vi "MemoryDialog.vi"(8 "Error In":errorcluster, 10 "Slot 1 Configuration":T1, 11 "Channel Patterns In":string[](array[string])) -> (0 "Error Out":errorcluster, 2 "Cancelled?":bool, 3 "Channel Patterns Out":string[](array[string]))   [LabVIEW 2012]
uses:
  SlotConfiguration.ctl
  BankConfiguration.ctl
  driver/Public/Controls/Slot.ctl
  libs/LV-Utilities/LV-Utilities.lvlib
  driver/Keithley-7001.lvlib
panel:
  out "Bank D Name":string
  out "Bank D Channel Names":string[](array[string])
  in  "Bank D Channel Enabled":bool[](array[boolean])
  out "Bank C Name":string
  out "Bank C Channel Names":string[](array[string])
  in  "Bank C Channel Enabled":bool[](array[boolean])
  out "Bank B Name":string
  out "Bank B Channel Names":string[](array[string])
  in  "Bank B Channel Enabled":bool[](array[boolean])=[FALSE, FALSE, FALSE, FALSE, FALSE, FALSE, FALSE, FALSE, FALSE, FALSE]
  out "Bank A Name":string
  out "Bank A Channel Names":string[](array[string])
  in  "Bank A Channel Enabled":bool[](array[boolean])=[FALSE, FALSE, FALSE, FALSE, FALSE, FALSE, FALSE, FALSE, FALSE, FALSE]
  in  "NEXT MEMORY LOCATION":bool
  in  "PREVIOUS MEMORY LOCATION":bool
  in  "Memory Location (1-100)":u8=1 min=1 max=100 step=1
  out "Channel Pattern":string
  in  "STORE":bool
  in  "RESET":bool
  in  "CANCEL":bool
  in  "DONE":bool
  # "CHANNELS"
  # "MEMORY"
  # "Location"
  # "Channel Pattern"
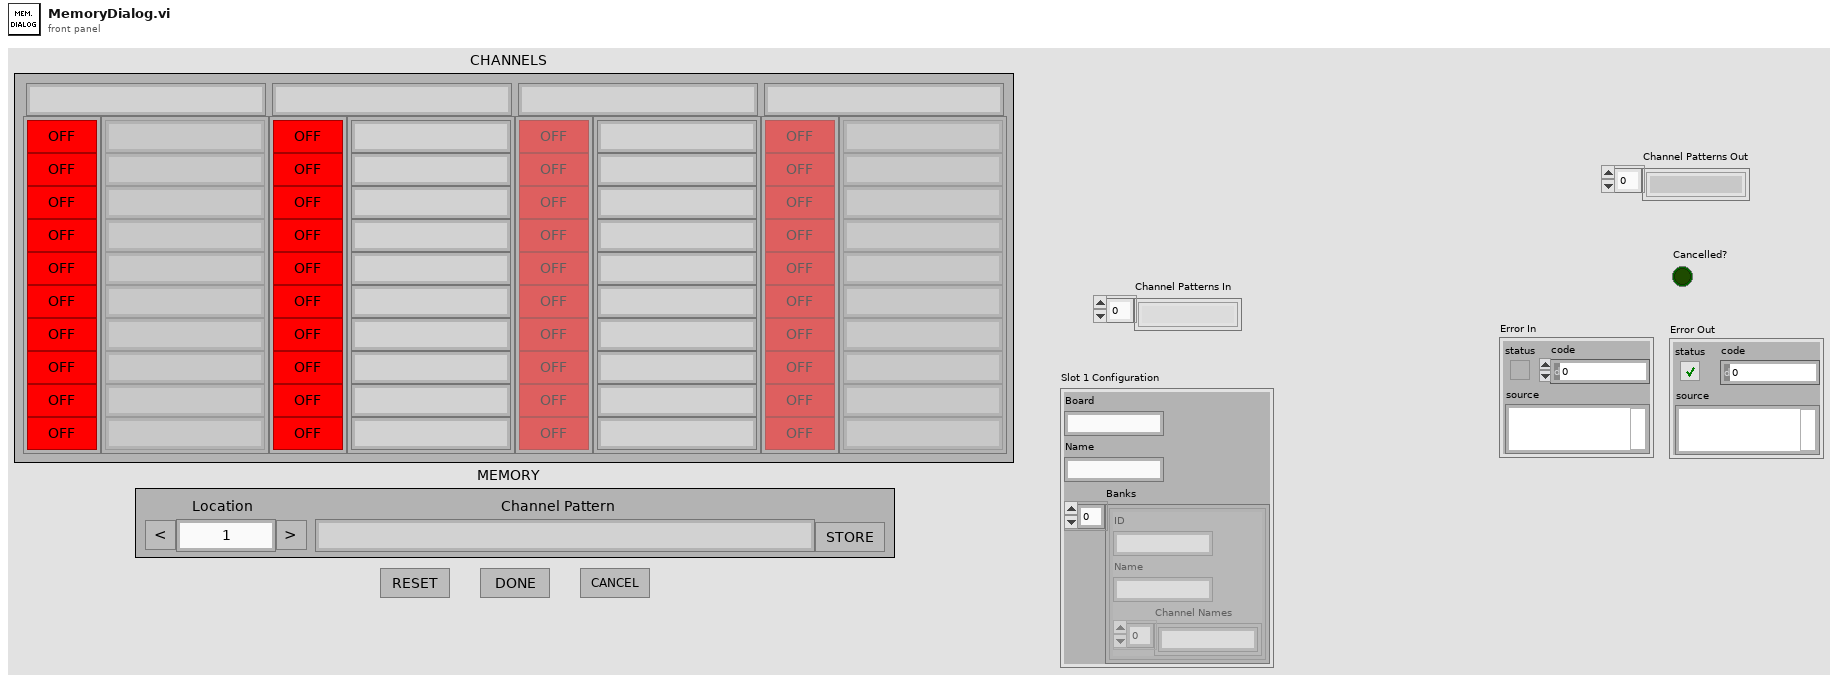
[diagram p1: front panel]
types:
  T1 = typedef "SlotConfiguration.ctl" = cluster{"Board":string, "Name":string, "Banks":T2[]}
  T2 = typedef "BankConfiguration.ctl" = cluster{"ID":string, "Name":string, "Channel Names":string[]}
  T3 = typedef "Keithley-7001.lvlib/Slot.ctl" = enum16{"Slot 1", "Slot 2"}
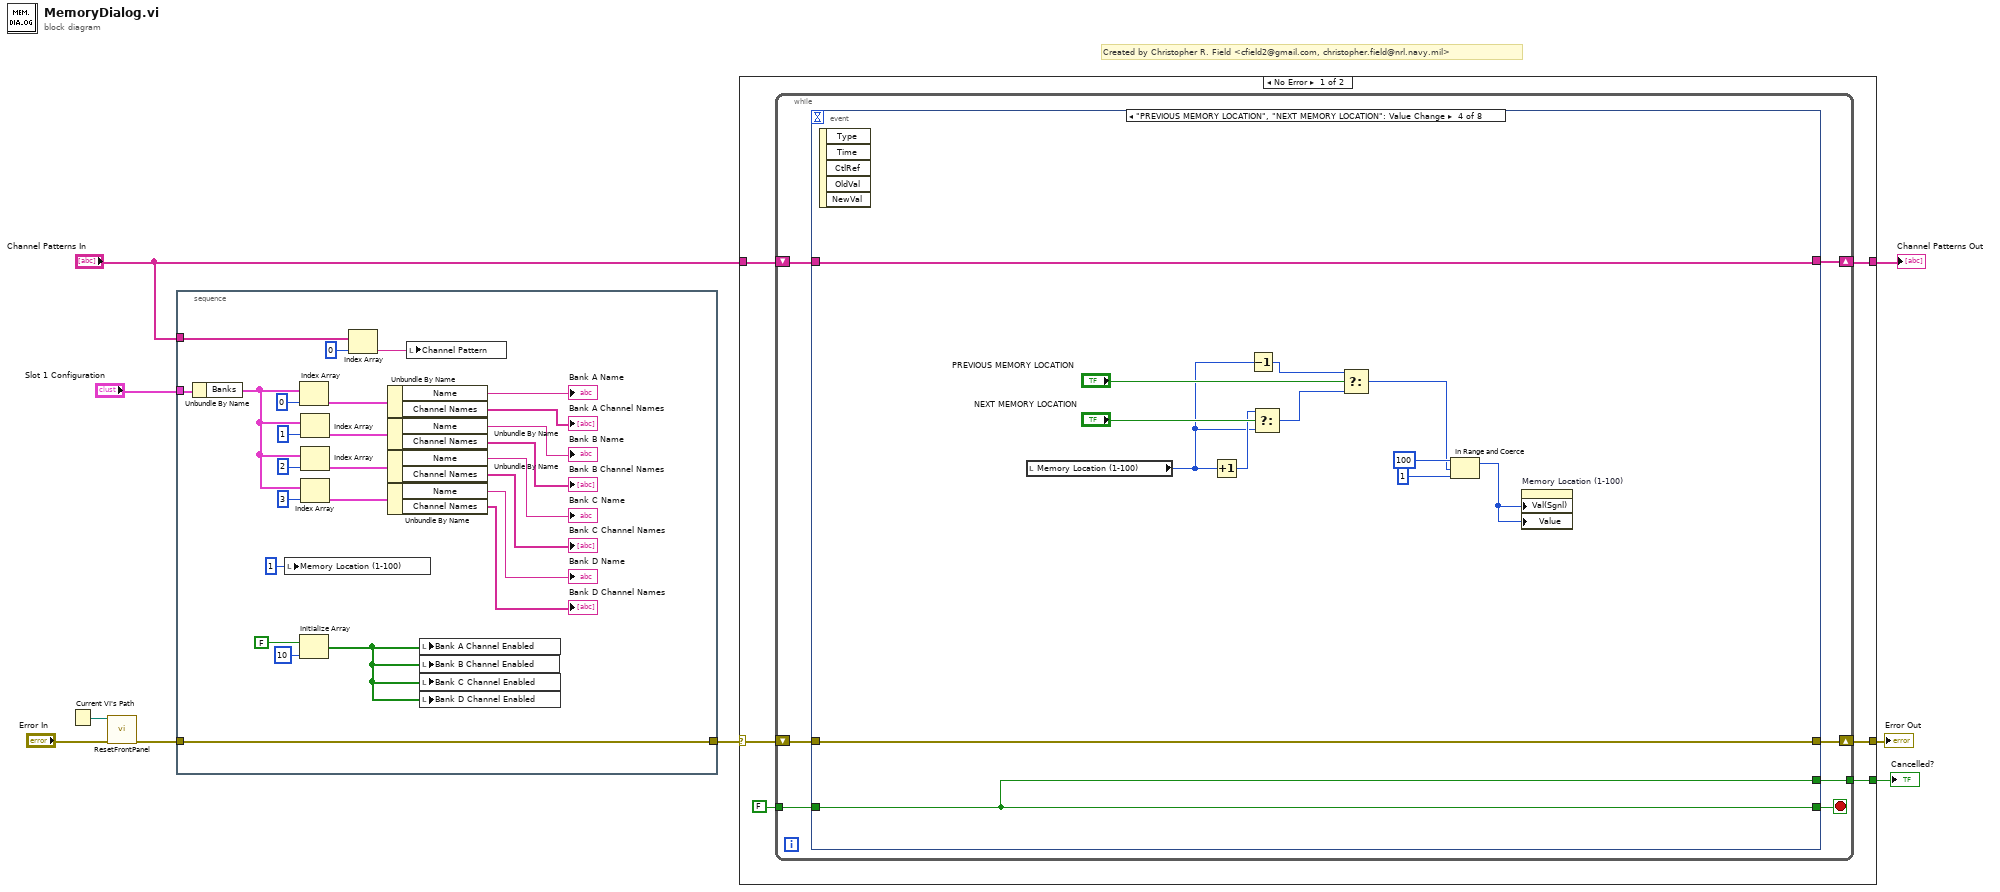
[diagram p0: block diagram]
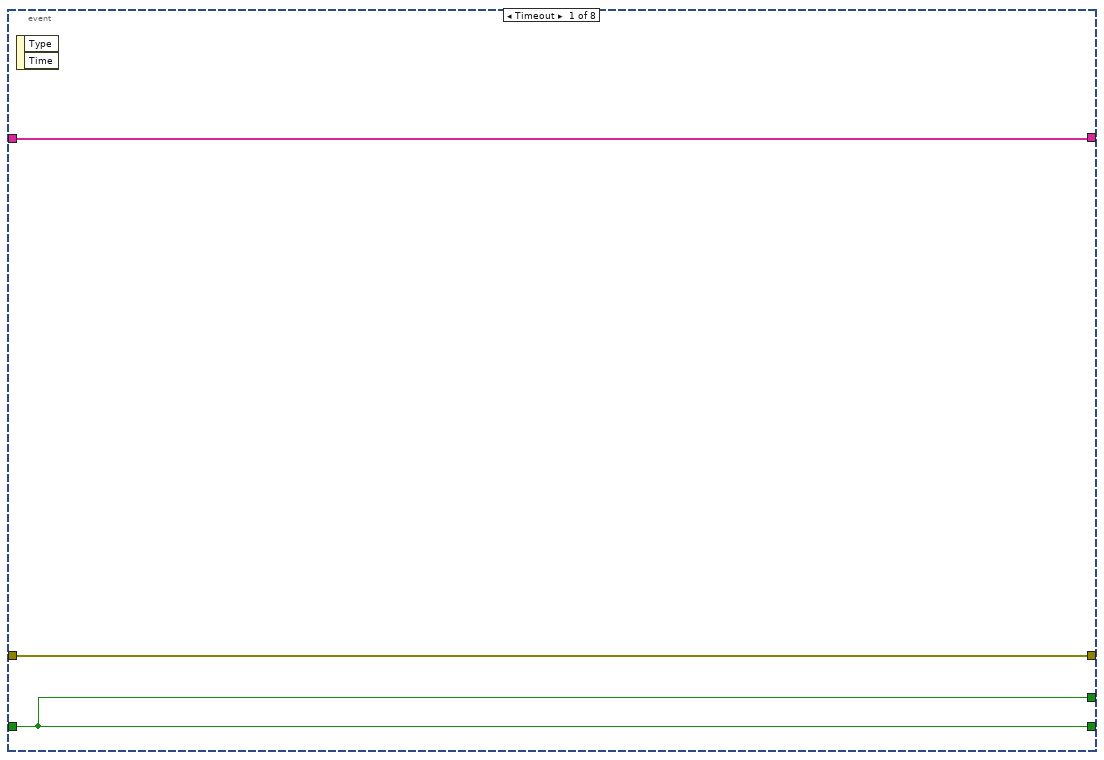
[diagram p2: hidden frame]
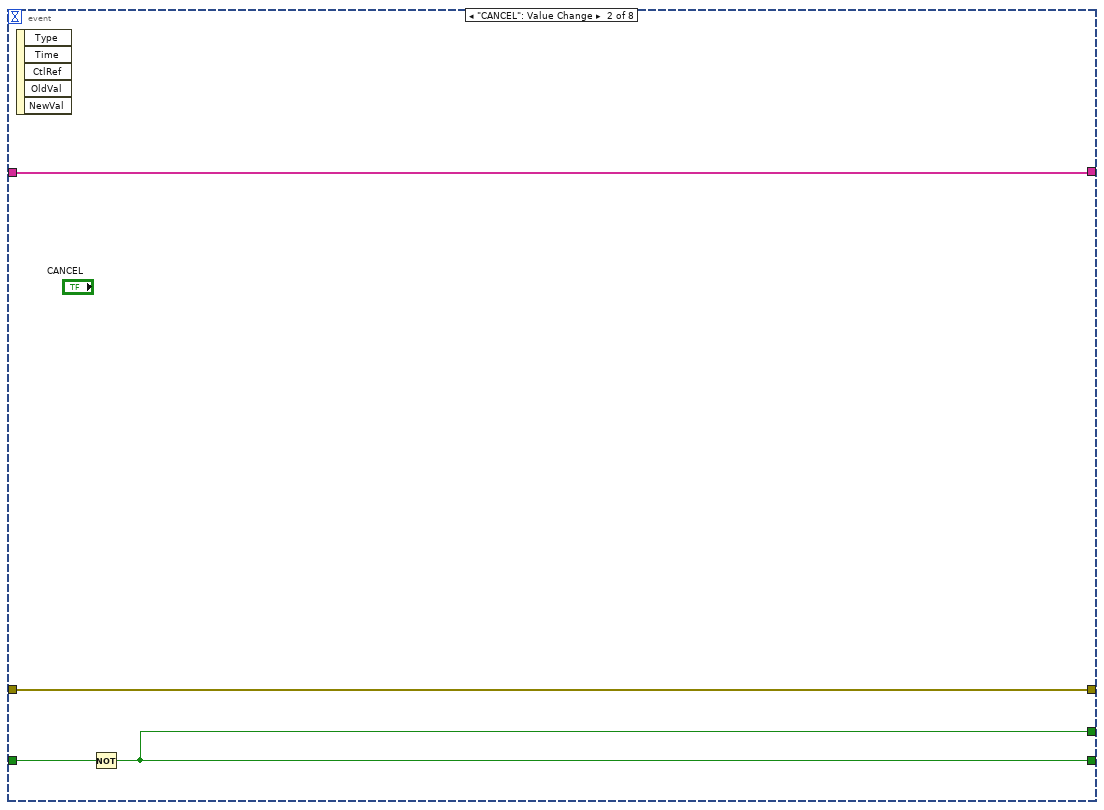
[diagram p3: hidden frame]
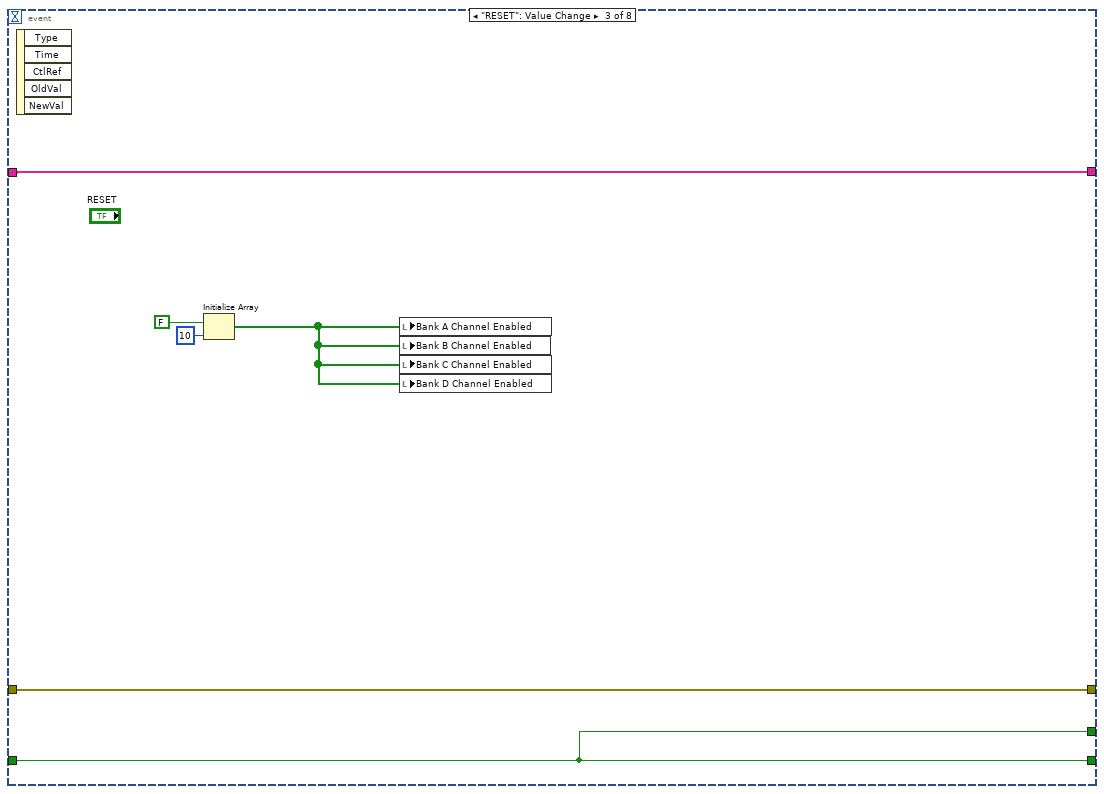
[diagram p4: hidden frame]
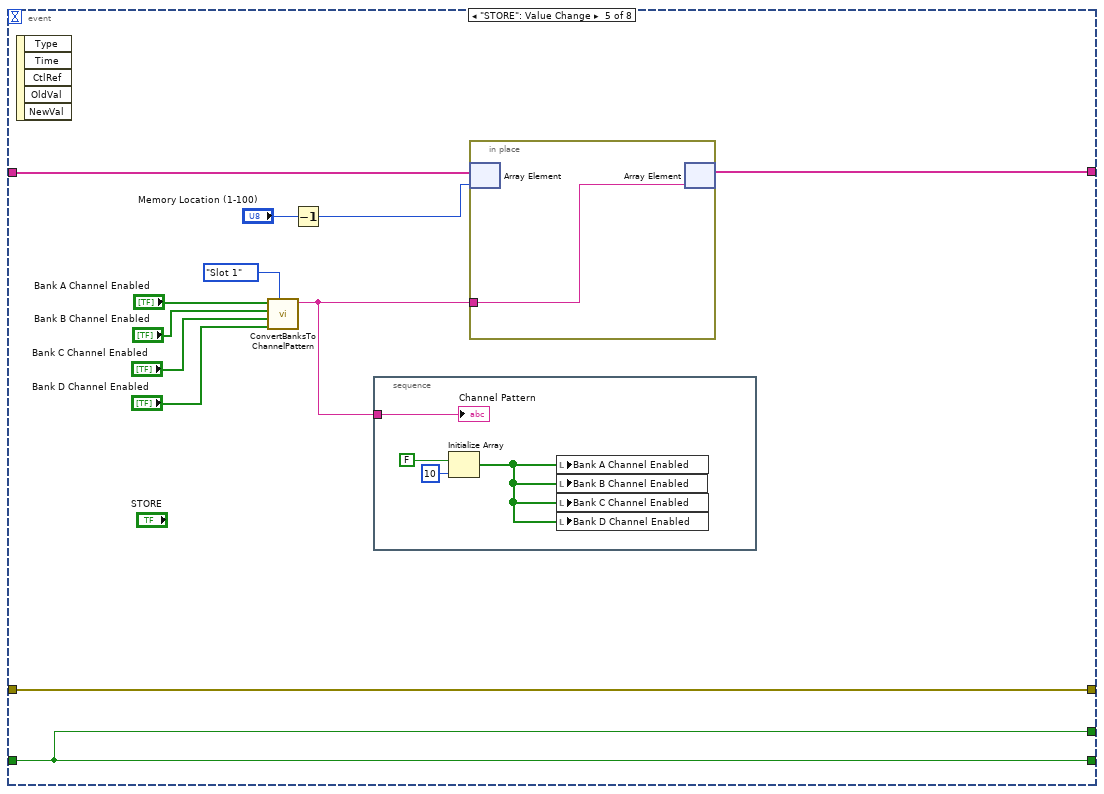
[diagram p5: hidden frame]
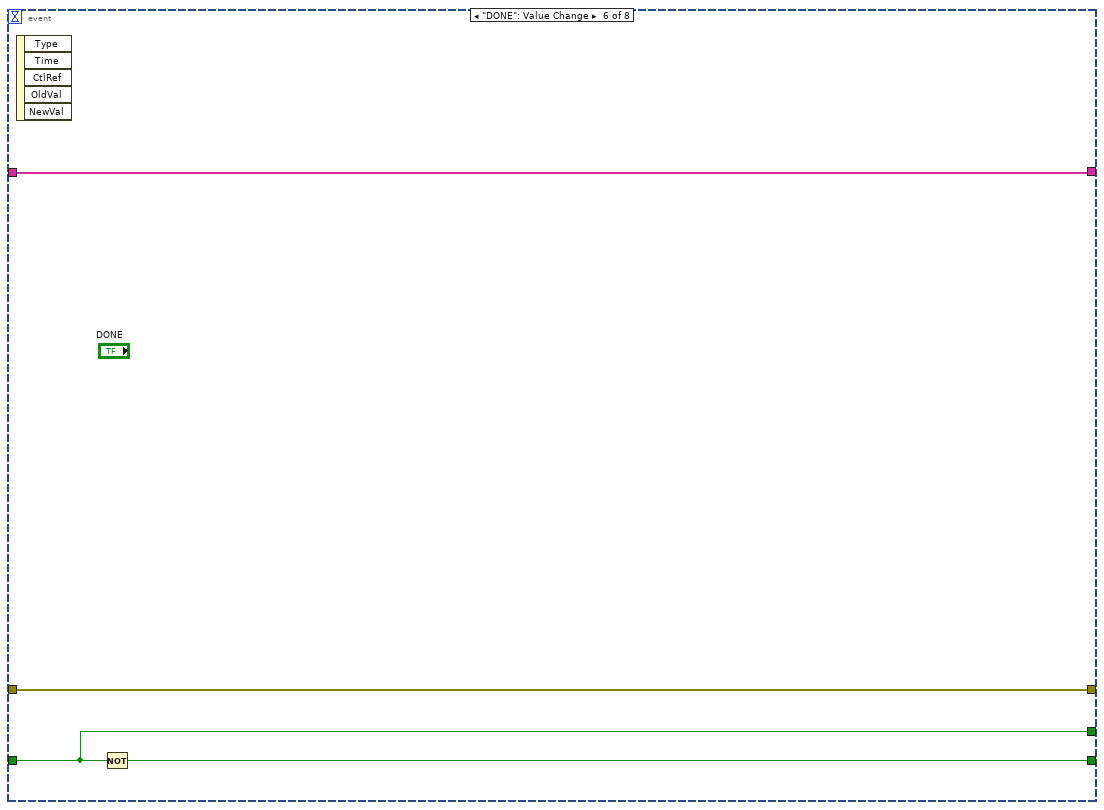
[diagram p6: hidden frame]
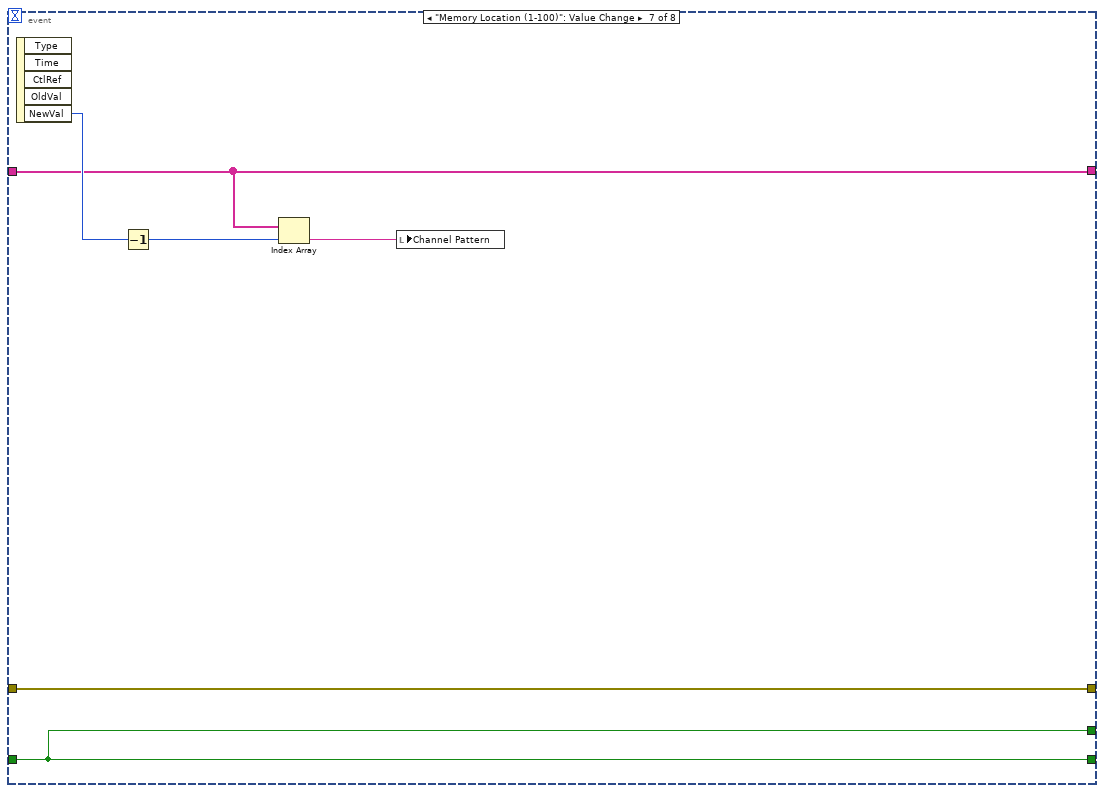
[diagram p7: hidden frame]
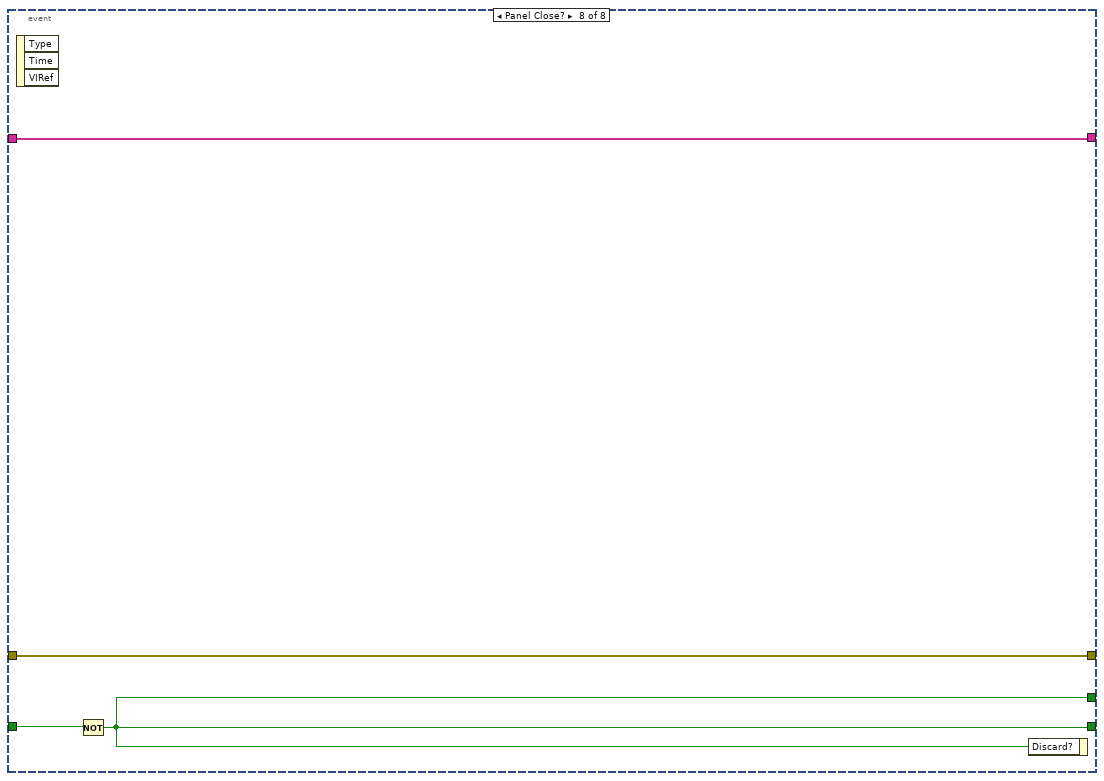
[diagram p8: hidden frame]
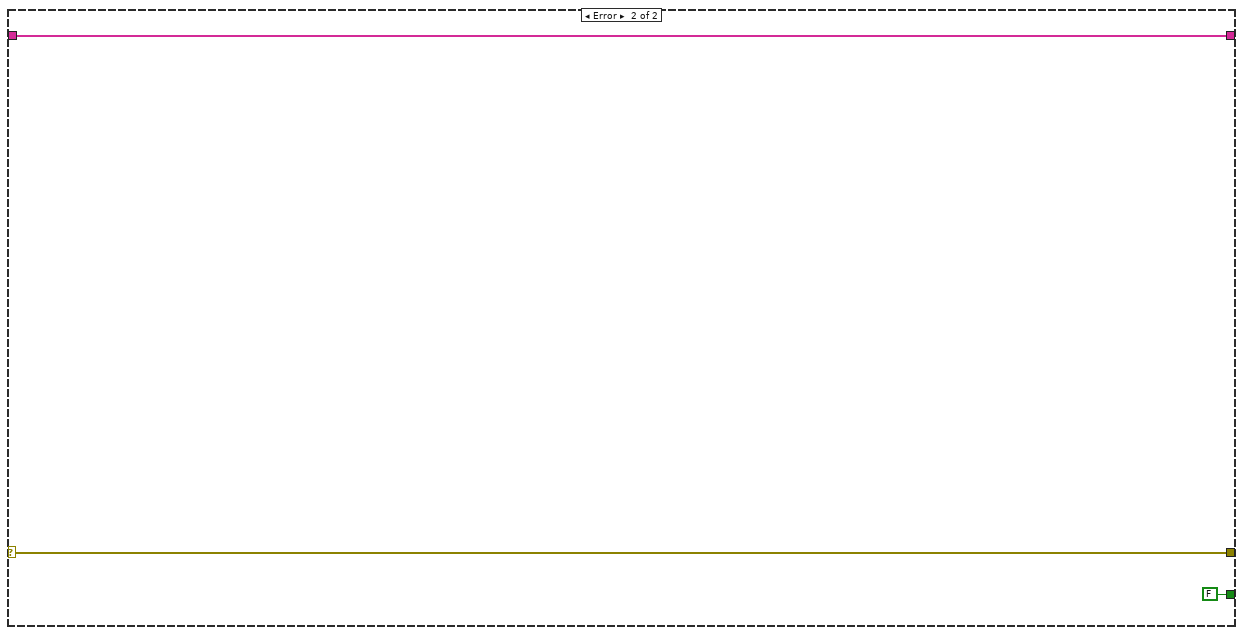
[diagram p9: hidden frame]
diagram:
  # "Created by Christopher R. Field <cfield2@gmail.com, christopher.field@nrl.navy.mil>"
  n1 = Current VI's Path() -> (path=w9:path)
  n2 = call "ResetFrontPanel.vi"("Error In"="Error In", "VI Path"=w9) -> ("Error Out"=w5:errorcluster)  [unwired: 9 in]
  n3 = stacked-sequence {
    tunnel: w5 -> [w35]
    tunnel: [w35] -> w4
    tunnel: "Channel Patterns In" -> [w30]
    tunnel: "Slot 1 Configuration" -> [w28]
    frame #0 {
      n4 = Unbundle By Name(w28) -> ("Banks"=w11:T2[])
      n5 = local write "Memory Location (1-100)"(u8 1 ("Memory Location (1-100)")) -> ()
      n6 = Index Array(array=w11, index=0) -> (element=w14:T2)
      n7 = Initialize Array(FALSE, 10 ("dimension size")) -> (w31:bool[])
      n8 = Index Array(array=w11, index=1) -> (element=w13:T2)
      n9 = Index Array(array=w11, index=2) -> (element=w12:T2)
      n10 = Index Array(array=w11, index=3) -> (element=w10:T2)
      n11 = Index Array(array=w30, index=0) -> (element=w29:string)
      n12 = Unbundle By Name(w14) -> ("Name"=→"Bank A Name":string, "Channel Names"=→"Bank A Channel Names":string[])
      n13 = Unbundle By Name(w13) -> ("Name"=→"Bank B Name":string, "Channel Names"=→"Bank B Channel Names":string[])
      n14 = Unbundle By Name(w12) -> ("Name"=→"Bank C Name":string, "Channel Names"=→"Bank C Channel Names":string[])
      n15 = Unbundle By Name(w10) -> ("Name"=→"Bank D Name":string, "Channel Names"=→"Bank D Channel Names":string[])
      n16 = local write "Channel Pattern"(w29) -> ()
      n17 = local write "Bank A Channel Enabled"(w31) -> ()
      n18 = local write "Bank B Channel Enabled"(w31) -> ()
      n19 = local write "Bank C Channel Enabled"(w31) -> ()
      n20 = local write "Bank D Channel Enabled"(w31) -> ()
    }
  }
  n21 = case shown="No Error" w4 {
    selector: w4 -> [w39 w108]
    tunnel: [w40 w108] -> w7
    tunnel: [w38 FALSE] -> w6
    tunnel: "Channel Patterns In" -> [w37 w106]
    tunnel: [w36 w106] -> w1
    frame No Error {
      n22 = while {
        tunnel: FALSE -> [w48]
        shift-right: [w45] -> w40
        shift-left: w39 -> [w46]
        tunnel: [w44] -> w38
        shift-right: [w42] -> w36
        shift-left: w37 -> [w43]
        stop <- w47 stop-if-true
        n23 = event shown="[3] \"PREVIOUS MEMORY LOCATION\", \"NEXT MEMORY LOCATION\": Value Change" {
          selector: _ -> [_ _ _ _ _ _ _ _]
          dyn-events: _ -> [_ _ _ _ _ _ _ _]
          timeout: _ -> [_ _ _ _ _ _ _ _]
          tunnel: w48 -> [w50 w54 w57 w72 w85 w93 w100 w104]
          tunnel: [w50 w53 w57 w72 w85 w94 w100 w103] -> w47
          tunnel: w46 -> [w51 w55 w58 w73 w86 w95 w101 w105]
          tunnel: [w51 w55 w58 w73 w86 w95 w101 w105] -> w45
          tunnel: [w50 w53 w57 w72 w85 w93 w100 w103] -> w44
          tunnel: w43 -> [w49 w52 w56 w74 w76 w92 w97 w102]
          tunnel: [w49 w52 w56 w74 w75 w92 w97 w102] -> w42
          event Timeout {
            n24 = event-data() -> ()  [unwired: 1 in, 2 out]
          }
          event "CANCEL": Value Change {
            n25 = event-data() -> ()  [unwired: 1 in, 5 out]
            n26 = Not(x=w54) -> (.not. x?=w53:bool)
          }
          event "RESET": Value Change {
            n27 = event-data() -> ()  [unwired: 1 in, 5 out]
            n28 = Initialize Array(FALSE, 10 ("dimension size")) -> (w59:bool[])
            n29 = local write "Bank A Channel Enabled"(w59) -> ()
            n30 = local write "Bank B Channel Enabled"(w59) -> ()
            n31 = local write "Bank C Channel Enabled"(w59) -> ()
            n32 = local write "Bank D Channel Enabled"(w59) -> ()
          }
          event "PREVIOUS MEMORY LOCATION", "NEXT MEMORY LOCATION": Value Change {
            n33 = event-data() -> ()  [unwired: 1 in, 5 out]
            n34 = local read "Memory Location (1-100)"() -> (w65:u8)
            n35 = Increment(x=w65) -> (x+1=w68:u8)
            n36 = Decrement(x=w65) -> (x-1=w64:u8)
            n37 = Select(t=w68, s="NEXT MEMORY LOCATION", f=w65) -> (s? t:f=w66:u8)
            n38 = Select(t=w64, s="PREVIOUS MEMORY LOCATION", f=w66) -> (s? t:f=w63:u8)
            n39 = In Range and Coerce(upper limit=u8 100, x=w63, lower limit=u8 1) -> (coerced(x)=w62:u8)  [unwired: 1 out]
            n40 = property on="Memory Location (1-100)" class="DigNum (strict)"("Val(Sgnl)"=w62, "Value"=w62) -> ()  [unwired: 2 in, 2 out]
          }
          event "STORE": Value Change {
            n41 = event-data() -> ()  [unwired: 1 in, 5 out]
            n42 = call "ConvertBanksToChannelPattern.vi"("Slot"=Slot."Slot 1", "Bank D Channel Enabled"="Bank D Channel Enabled", "Bank C Channel Enabled"="Bank C Channel Enabled", "Bank B Channel Enabled"="Bank B Channel Enabled", "Bank A Channel Enabled"="Bank A Channel Enabled") -> ("Channel Pattern"=w77:string)  [unwired: 6 in]
            n43 = Decrement(x="Memory Location (1-100)") -> (x-1=w82:u8)
            n44 = stacked-sequence {
              tunnel: w77 -> [w91]
              frame #0 {
                n45 = Initialize Array(FALSE, 10 ("dimension size")) -> (w88:bool[])
                n46 = local write "Bank A Channel Enabled"(w88) -> ()
                n47 = local write "Bank B Channel Enabled"(w88) -> ()
                n48 = local write "Bank C Channel Enabled"(w88) -> ()
                n49 = local write "Bank D Channel Enabled"(w88) -> ()
                "Channel Pattern" <- w91
              }
            }
            n50 = in-place {
              in-place-border: w77 -> [w87]
              n51 = in-place-array #1(w76, w82) -> ()  [unwired: 1 out]
              n52 = in-place-array #1(w87) -> (w75:string[])  [unwired: 1 out]
            }
          }
          event "DONE": Value Change {
            n53 = event-data() -> ()  [unwired: 1 in, 5 out]
            n54 = Not(x=w93) -> (.not. x?=w94:bool)
          }
          event "Memory Location (1-100)": Value Change {
            n55 = event-data() -> ("NewVal"=w99:u8)  [unwired: 1 in, 4 out]
            n56 = Decrement(x=w99) -> (x-1=w98:u8)
            n57 = Index Array(array=w97, index=w98) -> (element=w96:string)
            n58 = local write "Channel Pattern"(w96) -> ()
          }
          event Panel Close? {
            n59 = event-data() -> ()  [unwired: 1 in, 3 out]
            n60 = Not(x=w104) -> (.not. x?=w103:bool)
            n61 = event-data("Discard?"=w103) -> ()  [unwired: 1 in, 1 out]
          }
        }
      }
    }
    frame Error {
    }
  }
  "Error Out" <- w7
  "Cancelled?" <- w6
  "Channel Patterns Out" <- w1
